vi "C1G2_Assemble SelectQuery.vi"(7 "Sample Rate":dbl=10000000.0 format="%#_6p", 9 "Parameters Query":T2={"DR"=FALSE, "M"=1, "TRext (T=Pilot Tone)"=FALSE, "Sel"=1, "Session"=0, "Q"=0, "Target"=FALSE} {"Session" items=["S0", "S1", "S2", "S3"]; "Sel" items=["All", "All2", "~SL", "SL"]; "M" items=["M=1", "M=2", "M=4", "M=8"]}, 10 "Parameters Select":T3={"Target"=0, "Action"=0, "MemBank"=1, "truncate"=FALSE} {"MemBank" items=["00 RFU", "01 EPC", "10 TID", "11 User"]; "Action" items=["000", "001", "010", "011", "100", "101", "110", "111"]; "Target" items=["000 Inventoried (S0)", "001 Inventoried (S1)", "010 Inventoried (S2)", "011 Inventoried (S3)", "100 SL", "101 RFU", "110 RFU", "111 RFU"]}, 11 "Parameters Symbols":T1={"Tari"=2.5e-05, "PW"=0.5, "factor for \"1\" symbol"=0.5, "RTcal"=2.5, "TRcal"=2.5, "Delimiter"=1.25e-05} {"TRcal" min=1.1 max=3.0 step=0.1; "RTcal" min=2.5 max=3.0 step=0.1; "factor for \"1\" symbol" min=0.5 max=1.0 step=0.1; "PW" min=0.265 max=0.525 step=0.001; "Tari" format="%#_3p"}) -> (2 "Signal out":u8[](array[numeric]))   [LabVIEW 2015]
panel:
  out "All":i32
  out "CW":i32
  out "Sym0":i32
  out "Sym1":i32
  out "String Select CRC16":string="10000010000000000"
  out "String Select":string="10000010000000000"
  out "String Query CRC5":string="10000010000000000"
  out "Array":bool[](array[boolean])
  out "CRC-5":u8[](array[numeric])=[1, 0, 1, 1, 0] format="%0x"
  out "String Query":string="10000010000000000"
  out "0, 1":i16[](array[numeric])=[1, 0, 0, 0, 0, 0, 1, 0, 0, 0, 0, 0, 0, 0, 0, 0, 0]
  out "Symbols":i32=53374
  out "Digital Waveform":waveform(u8)(graph)={"t0"=timestamp(0 s since 1904-01-01), "dt"=1e-07, "Y"=array[53374 elements]}
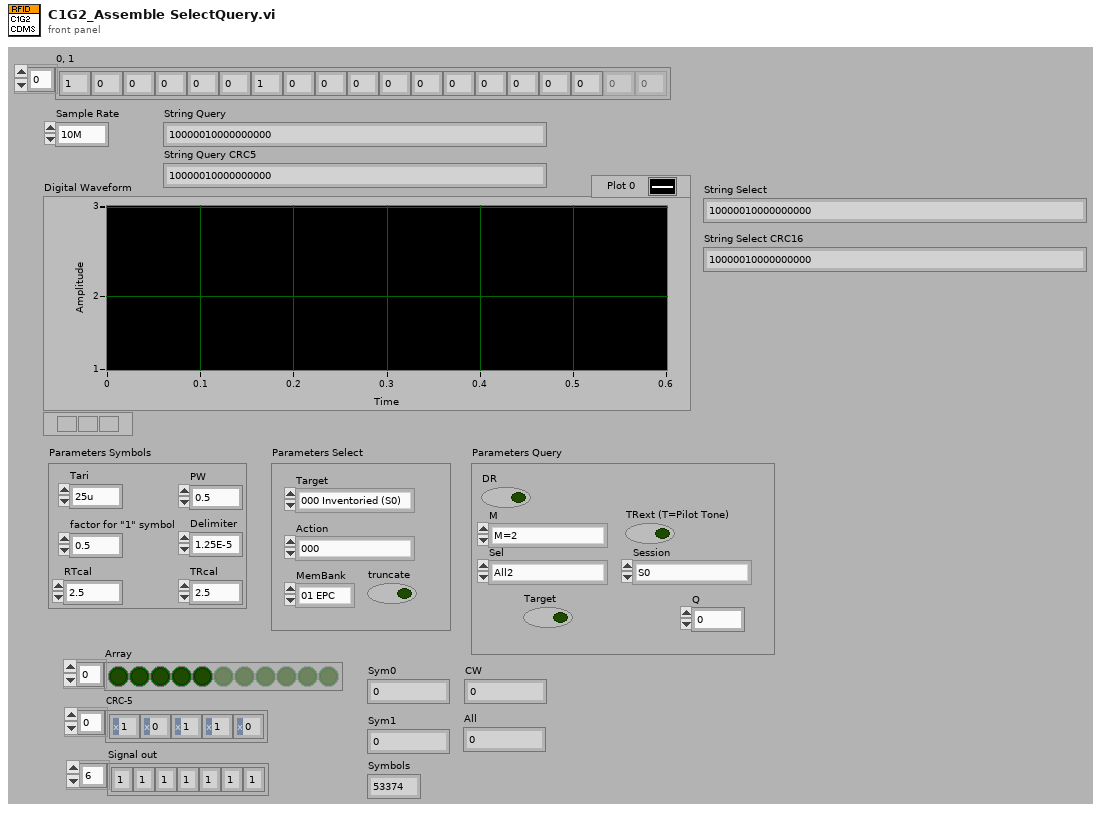
[diagram p1: front panel]
types:
  T1 = cluster{"Tari":dbl, "PW":dbl, "factor for \"1\" symbol":dbl, "RTcal":dbl, "TRcal":dbl, "Delimiter":dbl}
  T2 = cluster{"DR":bool, "M":u16, "TRext (T=Pilot Tone)":bool, "Sel":u16, "Session":u16, "Q":u8, "Target":bool}
  T3 = cluster{"Target":u16, "Action":u16, "MemBank":u16, "truncate":bool}
  T4 = typedef "C1G2_BasicsData.ctl" = cluster{"Symbol \"0\"":u8[], "Symbol \"1\"":u8[], "RT Preamble":u8[], "RT Frame Sync":u8[], "Sample Rate":dbl, "LOW-Pulse":u8[], "HIGH-Pulse":u8[], "RT cal":u8[]}
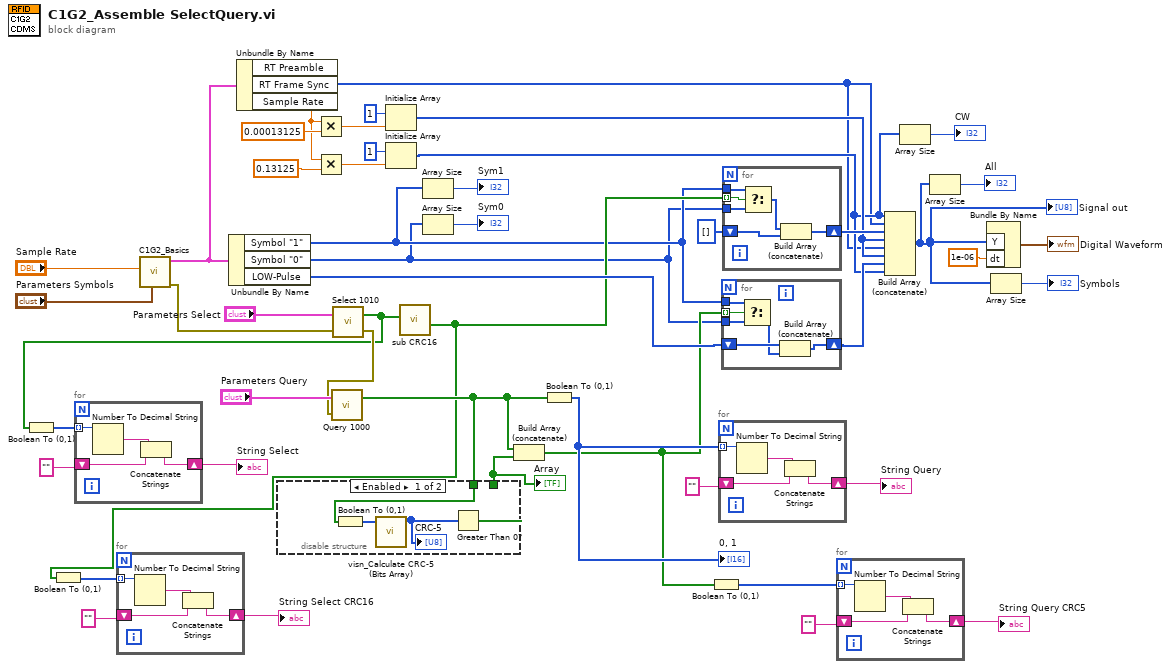
[diagram p0: block diagram]
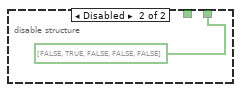
[diagram p2: hidden frame]
diagram:
  n1 = call "C1G2_Basics.vi"("Parameters Symbols"="Parameters Symbols", "Sample Rate"="Sample Rate") -> ("error out"=w23:errorcluster, "Basic Components"=w30:T4)  [unwired: 8 in]
  n2 = Unbundle By Name(w30) -> ("Symbol \"1\""=w8:u8[], "Symbol \"0\""=w6:u8[], "LOW-Pulse"=w29:u8[])
  n3 = Unbundle By Name(w30) -> ("RT Frame Sync"=w1:u8[], "Sample Rate"=w34:dbl)  [unwired: 1 out]
  n4 = Multiply(x=w34, y=0.00013125 ("Pause length /s")) -> (x*y=w40:dbl)
  n5 = Multiply(x=w34, y=0.13125 ("Pause length /s")) -> (x*y=w36:dbl)
  n6 = call "Select 1010.vi"("error in (no error)"=w23, "Parameters Select"="Parameters Select") -> ("error out"=w22:errorcluster, "Array"=w14:bool[])
  n7 = Boolean To (0,1)(Boolean=w14) -> (0, 1=w15:i16[])
  n8 = for {
    tunnel: w15 -> [w52] mode=indexing
    shift-right: [w49] -> w16
    shift-left: "" -> [w50]
    n9 = Number To Decimal String(number=w52) -> (decimal integer string=w51:string)  [unwired: 1 in]
    n10 = Concatenate Strings(w50, w51) -> (w49:string)
  }
  "String Select" <- w16
  n11 = call "Query 1000.vi"("error in (no error)"=w22, "Parameters Query"="Parameters Query") -> ("Array"=w25:bool[])  [unwired: 1 out]
  n12 = disable-structure shown="Enabled" {
    disable-tunnel: w25 -> [w55 _]
    disable-tunnel: [w53 bool[] [FALSE, TRUE, FALSE, FALSE, FALSE]] -> w24
    frame Enabled {
      n13 = Boolean To (0,1)(Boolean=w55) -> (0, 1=w56:i16[])
      n14 = call "visn_Calculate CRC-5 (Bits Array).vi"("Bits Array"=w56) -> ("CRC-5"=w54:u8[])  [unwired: 10 in]
      "CRC-5" <- w54
      n15 = Greater Than 0?(x=w54) -> (x > 0?=w53:bool[])
    }
    frame Disabled {
    }
  }
  "Array" <- w24
  n16 = Initialize Array(u8 1 ("element"), w40) -> (w32:u8[])
  n17 = Initialize Array(u8 1 ("element"), w36) -> (w4:u8[])
  n18 = call "sub CRC16.vi"("Data in"=w14) -> ("Data + CRC 16"=w10:bool[])  [unwired: 5 in, 1 out]
  n19 = Boolean To (0,1)(Boolean=w10) -> (0, 1=w11:i16[])
  n20 = for {
    tunnel: w11 -> [w61] mode=indexing
    shift-right: [w58] -> w12
    shift-left: "" -> [w59]
    n21 = Number To Decimal String(number=w61) -> (decimal integer string=w60:string)  [unwired: 1 in]
    n22 = Concatenate Strings(w59, w60) -> (w58:string)
  }
  "String Select CRC16" <- w12
  n23 = Array Size(array=w8) -> (size(s)=→"Sym1":i32)
  n24 = Array Size(array=w6) -> (size(s)=→"Sym0":i32)
  n25 = Build Array (concatenate)(w25, w24) -> (w18:bool[])
  n26 = Boolean To (0,1)(Boolean=w25) -> (0, 1=w28:i16[])
  "0, 1" <- w28
  n27 = Boolean To (0,1)(Boolean=w18) -> (0, 1=w19:i16[])
  n28 = for {
    tunnel: w28 -> [w65] mode=indexing
    shift-right: [w62] -> w26
    shift-left: "" -> [w63]
    n29 = Number To Decimal String(number=w65) -> (decimal integer string=w64:string)  [unwired: 1 in]
    n30 = Concatenate Strings(w63, w64) -> (w62:string)
  }
  "String Query" <- w26
  n31 = for {
    tunnel: w18 -> [w71] mode=indexing
    tunnel: w6 -> [w69]
    tunnel: w8 -> [w70]
    shift-right: [w68] -> w31
    shift-left: w29 -> [w67]
    n32 = Select(t=w70, s=w71, f=w69) -> (s? t:f=w66:u8[])
    n33 = Build Array (concatenate)(w67, w66) -> (w68:u8[])
  }
  n34 = for {
    tunnel: w10 -> [w77] mode=indexing
    tunnel: w6 -> [w75]
    tunnel: w8 -> [w76]
    shift-right: [w74] -> w41
    shift-left: u8[] [] ("s? t:f") -> [w73]
    n35 = Select(t=w76, s=w77, f=w75) -> (s? t:f=w72:u8[])
    n36 = Build Array (concatenate)(w72, w73) -> (w74:u8[])
  }
  n37 = for {
    tunnel: w19 -> [w81] mode=indexing
    shift-right: [w78] -> w20
    shift-left: "" -> [w79]
    n38 = Number To Decimal String(number=w81) -> (decimal integer string=w80:string)  [unwired: 1 in]
    n39 = Concatenate Strings(w79, w80) -> (w78:string)
  }
  "String Query CRC5" <- w20
  n40 = Build Array (concatenate)(w4, w1, w41, w32, w1, w32, w31, w4) -> (w2:u8[])
  "Signal out" <- w2
  n41 = Array Size(array=w4) -> (size(s)=→"CW":i32)
  n42 = Array Size(array=w2) -> (size(s)=→"All":i32)
  n43 = Bundle By Name("Y"=w2, "dt"=1e-06) -> (→"Digital Waveform":waveform(u8))  [unwired: 1 in]
  n44 = Array Size(array=w2) -> (size(s)=→"Symbols":i32)
